vi "expt overnight automator set coils and save - arb coil patterns.vi"() -> ()   [LabVIEW 2018]
panel:
  in  "Save?":bool=TRUE
  in  "Field (Gauss)":u16(ring)=1 items=["9G"=1, "14G"=2]
  out "num coil iters done":i32
  out "total pos sweeps":i32
  out "total neg sweeps":i32
  in  "?":bool
  out "numSweeps list":i64[](array[numeric])=[10, 20, 10, 10, 20, 10]
  out "polarity list":i64[](array[numeric])=[-1, 1, -1, 1, -1, 1]
  in  "polarity pattern file":path=path "D:/rogers_data/GRA95229/115/thermal/115_s2_NWsulfide/TT_143C/P.txt"
  in  "num coil iterations":i32=2
  out "freq list (Hz)":dbl[](array[numeric])
  out "+Z current out (mA)":dbl=-975.0
  out "+Y current out (mA)":dbl=-1500.0
  out "+X current out (mA)":dbl=-20.0
  out "-Z current out (mA)":dbl=-975.0
  out "-Y current out (mA)":dbl=-1500.0
  out "-X current out (mA)":dbl=-20.0
  out "header cluster":T1
  in  "filename (adds .mat)":string="run_"
  in  "path":path=path "D:/rogers_data/GRA95229/115/thermal/115_s2_NWsulfide/TT_143C"
  out "coil polarity":bool=TRUE
  out "img data stack pos":dbl[][](array[numeric])
  in  "Height":i64(slide)=1200 min=0 max=1200 step=4 scale=0.0..1200.0
  in  "Width":i64(slide)=1920 min=0 max=1920 step=4 scale=0.0..1920.0
  out "img data stack neg":dbl[][](array[numeric])
  in  "freq range":T2(ring)=enum."Both ranges"
  in  "num freqs":i32=51
  out "set later end time!":bool
  out "current time":timestamp
  in  "end time (>current time)":timestamp=timestamp(3667924096.6668215 s since 1904-01-01)
  # "Coil parameters"
  # "Set time"
  # "Coil polarity"
  # "ODMR parameters"
  # "File setup"
  # "Camera parameters"
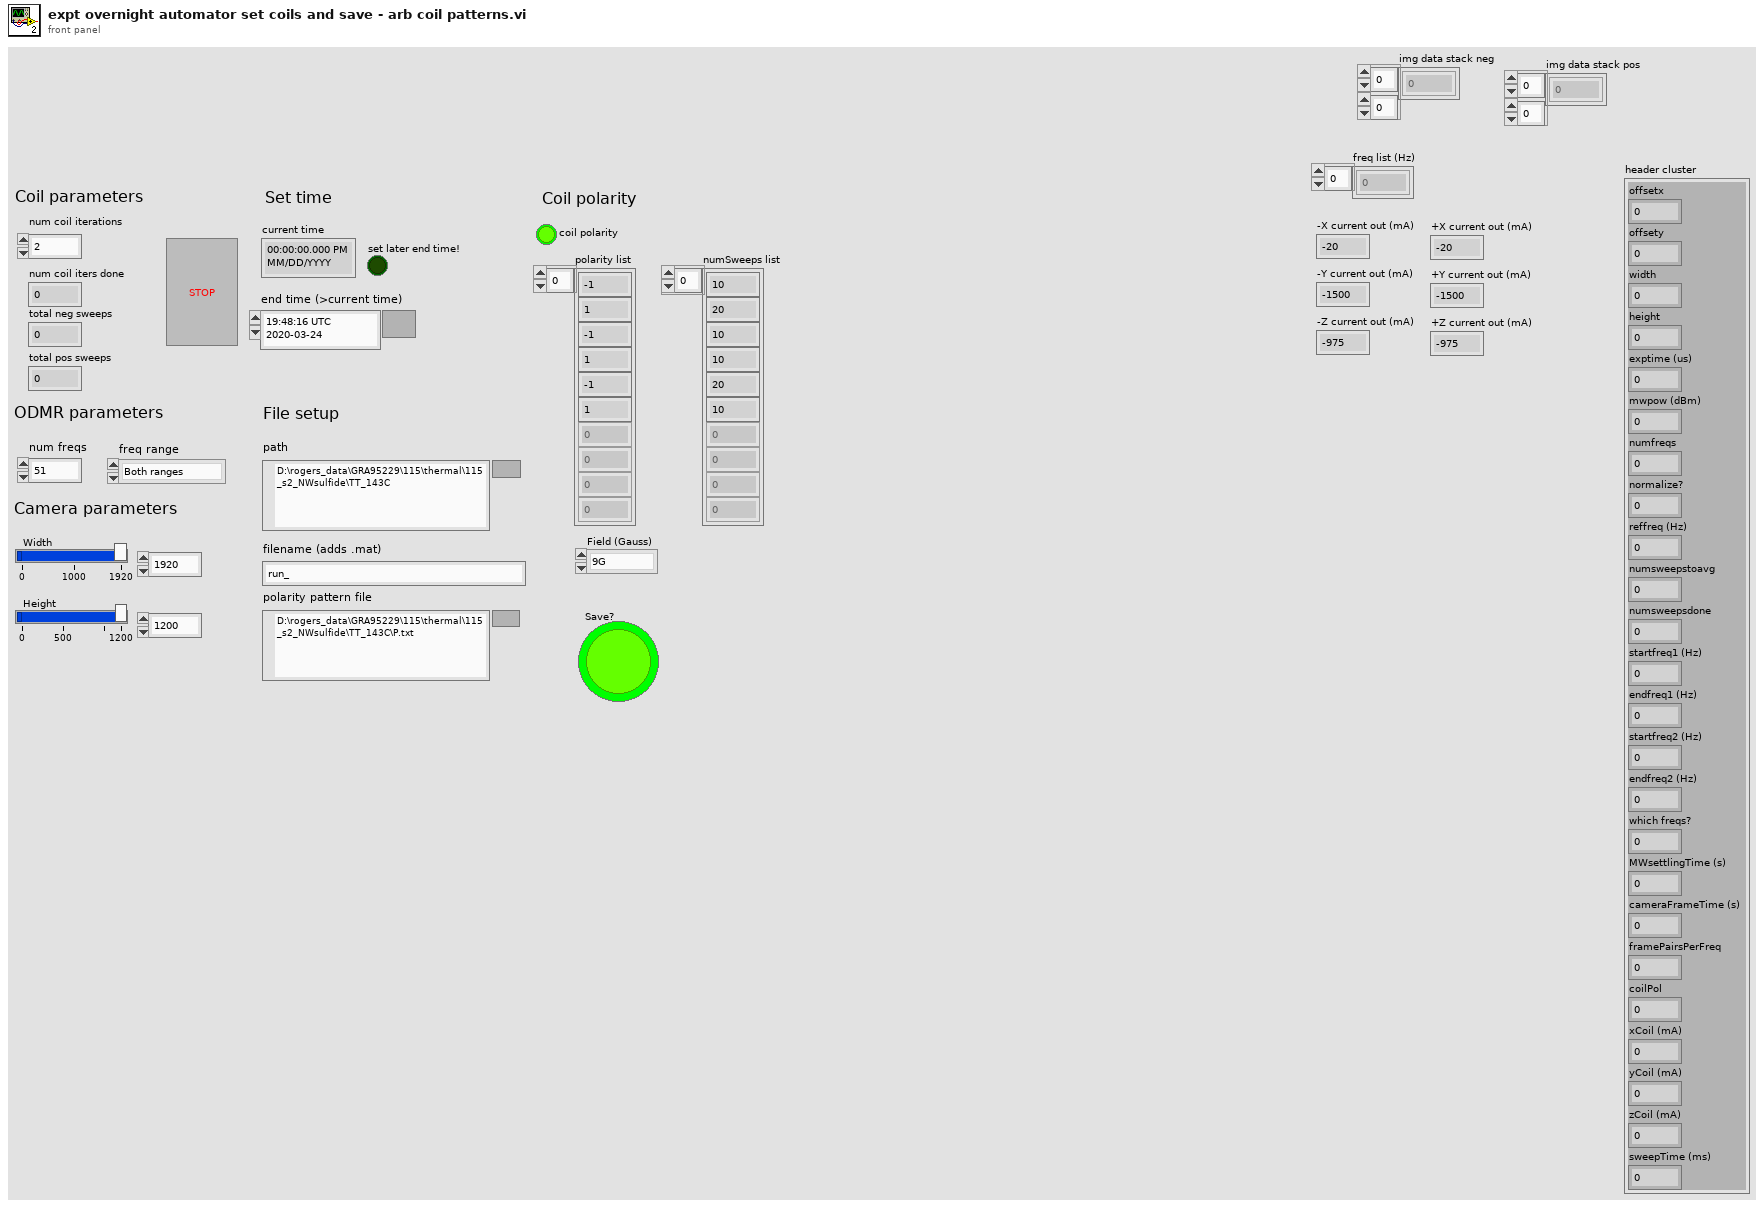
[diagram p1: front panel]
types:
  T1 = cluster{"offsetx":i64, "offsety":i64, "width":i64, "height":i64, "exptime (us)":dbl, "mwpow (dBm)":dbl, "numfreqs":i32, "normalize?":i32, "reffreq (Hz)":dbl, "numsweepstoavg":i32, "numsweepsdone":i32, "startfreq1 (Hz)":dbl, "endfreq1 (Hz)":dbl, "startfreq2 (Hz)":dbl, "endfreq2 (Hz)":dbl, "which freqs?":i32, "MWsettlingTime (s)":dbl, "cameraFrameTime (s)":dbl, "framePairsPerFreq":i32, "coilPol":i32, "xCoil (mA)":dbl, "yCoil (mA)":dbl, "zCoil (mA)":dbl, "sweepTime (ms)":i32}
  T2 = enum16{"Lower range", "Upper range", "Both ranges"}
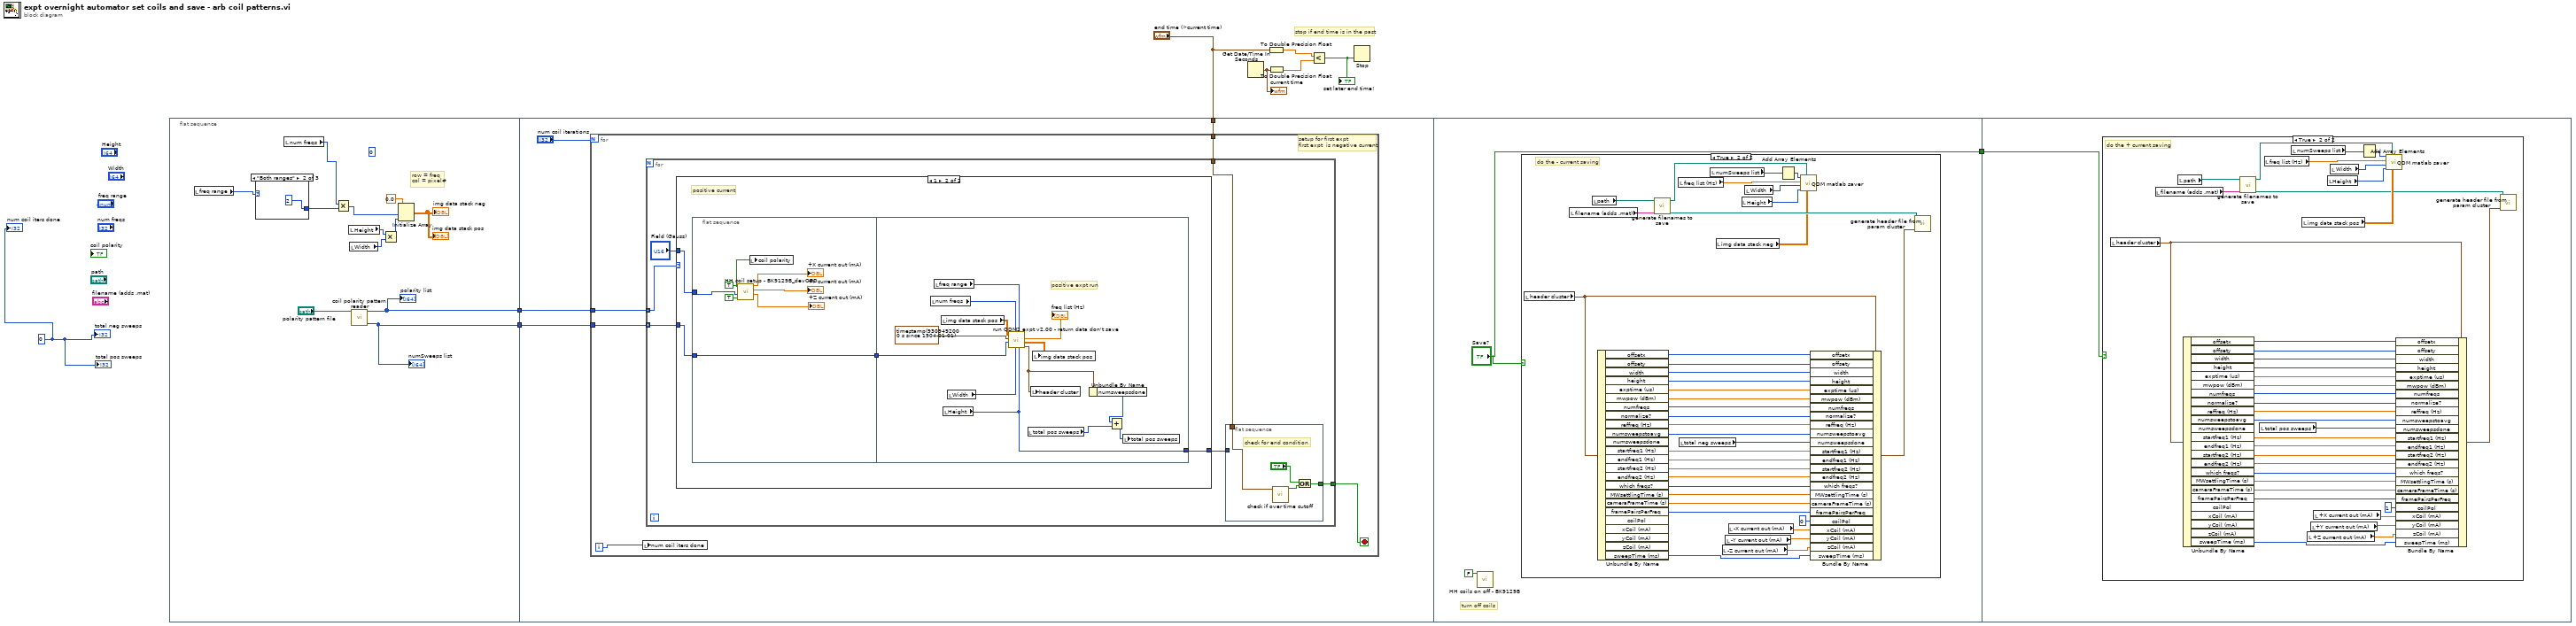
[diagram p0: block diagram]
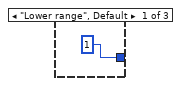
[diagram p2: hidden frame]
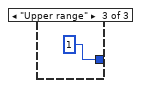
[diagram p3: hidden frame]
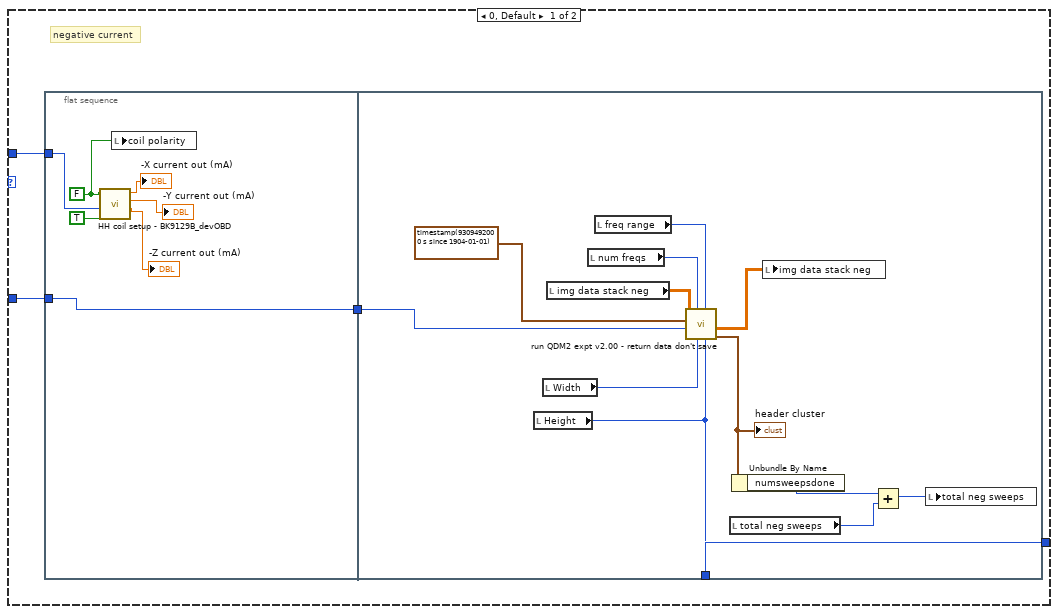
[diagram p4: hidden frame]
diagram:
  w2 = 0
  # "stop if end time is in the past"
  n1 = flat-sequence {
    tunnel: [w11] -> w9
    tunnel: [w10] -> w8
    tunnel: w9 -> [w28]
    tunnel: w8 -> [w27]
    tunnel: "end time (>current time)" -> [w25]
    tunnel: ["Save?"] -> w1
    tunnel: w1 -> [w129]
    frame #0 {
      (unwired) 0 ("1st half sweeps")
      # "row = freq\ncol = pixel#"
      n2 = local read "freq range"() -> (w13:T2)
      n3 = case shown="\"Both ranges\"" w13 {
        tunnel: [1 ("numFreqs") 2 ("numFreqs") 1 ("numFreqs")] -> w16
        frame "Lower range", Default {
        }
        frame "Both ranges" {
        }
        frame "Upper range" {
        }
      }
      n4 = local read "num freqs"() -> (w14:i32)
      n5 = Multiply(x=w14, y=w16) -> (x*y=w15:i32)
      n6 = local read "Height"() -> (w21:i64)
      n7 = local read "Width"() -> (w20:i64)
      n8 = call "coil polarity pattern reader.vi"("polarity pattern file"="polarity pattern file") -> ("numSweeps list"=w10:i64[], "polarity list"=w11:i64[])  [unwired: 9 in]
      "polarity list" <- w11
      "numSweeps list" <- w10
      n9 = Multiply(x=w21, y=w20) -> (x*y=w19:i64)
      n10 = Initialize Array(0.0 ("element"), w15, w19) -> (→"img data stack pos" →"img data stack neg":dbl[][])
    }
    frame #1 {
      n11 = for {
        N: "num coil iterations" -> [_]
        tunnel: w28 -> [w33]
        tunnel: w27 -> [w32]
        tunnel: w25 -> [w30]
        i -> [w29]
        stop <- w31 stop-if-true
        # "setup for first expt\nfirst expt  is negative current"
        n12 = local write "num coil iters done"(w29) -> ()
        n13 = for {
          tunnel: w33 -> [w39] mode=indexing
          tunnel: w32 -> [w38] mode=indexing
          tunnel: [w36] -> w31
          tunnel: w30 -> [w35]
          n14 = case shown="1" w39 {
            tunnel: w38 -> [w46 w70]
            tunnel: [w45 w68] -> w37
            tunnel: "Field (Gauss)" -> [w44 w67]
            frame 0, Default {
              # "negative current"
              n15 = flat-sequence {
                tunnel: [w54] -> w47
                tunnel: w46 -> [w54]
                tunnel: w44 -> [w48]
                tunnel: w47 -> [w61]
                tunnel: [w59] -> w45
                frame #0 {
                  w53 = FALSE ("coil polarity")
                  n16 = call "HH coil setup - BK9129B_devOBD.VI"("setup enabled?"=TRUE, "number"=w48, "coil polarity"=w53) -> ("Z current out (mA)"=→"-Z current out (mA)":dbl, "Y current out (mA)"=→"-Y current out (mA)":dbl, "X current out (mA)"=→"-X current out (mA)":dbl)  [unwired: 6 in]
                  n17 = local write "coil polarity"(w53) -> ()
                }
                frame #1 {
                  n18 = local read "Height"() -> (w59:i64)
                  n19 = local read "Width"() -> (w64:i64)
                  n20 = local read "img data stack neg"() -> (w62:dbl[][])
                  n21 = local read "num freqs"() -> (w66:i32)
                  n22 = local read "freq range"() -> (w65:T2)
                  n23 = call "run QDM2 expt v2.00 - return data don't save.vi"("Height"=w59, "which freqs?"=w65, "Width"=w64, "numFreqs"=w66, "num sweeps to avg"=w61, "cutoff time"=timestamp(9309492000 s since 1904-01-01), "img data stack Input"=w62) -> ("header cluster"=w58:T1, "img data stack Return"=w63:dbl[][])  [unwired: 1 in, 2 out]
                  "header cluster" <- w58
                  n24 = local read "total neg sweeps"() -> (w56:i32)
                  n25 = Unbundle By Name(w58) -> ("numsweepsdone"=w57:i32)
                  n26 = local write "img data stack neg"(w63) -> ()
                  n27 = Add(x=w57, y=w56) -> (x+y=w55:i32)
                  n28 = local write "total neg sweeps"(w55) -> ()
                }
              }
            }
            frame 1 {
              # "positive current"
              n29 = flat-sequence {
                tunnel: w70 -> [w72]
                tunnel: [w72] -> w69
                tunnel: w67 -> [w71]
                tunnel: w69 -> [w83]
                tunnel: [w82] -> w68
                frame #0 {
                  w73 = TRUE ("coil polarity")
                  n30 = call "HH coil setup - BK9129B_devOBD.VI"("setup enabled?"=TRUE, "number"=w71, "coil polarity"=w73) -> ("Z current out (mA)"=→"+Z current out (mA)":dbl, "Y current out (mA)"=→"+Y current out (mA)":dbl, "X current out (mA)"=→"+X current out (mA)":dbl)  [unwired: 6 in]
                  n31 = local write "coil polarity"(w73) -> ()
                }
                frame #1 {
                  # "positive expt run"
                  n32 = local read "num freqs"() -> (w90:i32)
                  n33 = local read "freq range"() -> (w89:T2)
                  n34 = local read "img data stack pos"() -> (w85:dbl[][])
                  n35 = local read "Height"() -> (w82:i64)
                  n36 = local read "Width"() -> (w88:i64)
                  n37 = call "run QDM2 expt v2.00 - return data don't save.vi"("Height"=w82, "which freqs?"=w89, "Width"=w88, "numFreqs"=w90, "num sweeps to avg"=w83, "cutoff time"=timestamp(9309492000 s since 1904-01-01), "img data stack Input"=w85) -> ("header cluster"=w81:T1, "img data stack Return"=w86:dbl[][], "freq list (Hz)"=→"freq list (Hz)":dbl[])  [unwired: 1 in, 1 out]
                  n38 = local read "total pos sweeps"() -> (w79:i32)
                  n39 = local write "header cluster"(w81) -> ()
                  n40 = local write "img data stack pos"(w86) -> ()
                  n41 = Unbundle By Name(w81) -> ("numsweepsdone"=w80:i32)
                  n42 = Add(x=w80, y=w79) -> (x+y=w78:i32)
                  n43 = local write "total pos sweeps"(w78) -> ()
                }
              }
            }
          }
          n44 = flat-sequence {
            tunnel: w37 -> [_]
            tunnel: [w41] -> w36
            tunnel: w35 -> [w40]
            frame #0 {
              # "check for end condition"
              n45 = call "check if over time cutoff.vi"("cutoff time"=w40) -> ("past due?"=w42:bool)  [unwired: 10 in]
              n46 = Or(x="?", y=w42) -> (x .or. y?=w41:bool)
            }
          }
        }
      }
    }
    frame #2 {
      # "turn off coils"
      n47 = call "HH coils on off - BK9129B.VI"("coils on?"=FALSE) -> ()  [unwired: 11 in]
      n48 = case shown="True" "Save?" {
        frame False {
        }
        frame True {
          # "do the - current saving"
          n49 = local read "header cluster"() -> (w103:T1)
          n50 = local read "filename (adds .mat)"() -> (w127:string)
          n51 = local read "path"() -> (w128:path)
          n52 = Unbundle By Name(w103) -> ("offsetx"=w104:i64, "offsety"=w105:i64, "width"=w106:i64, "height"=w107:i64, "exptime (us)"=w108:dbl, "mwpow (dBm)"=w109:dbl, "numfreqs"=w110:i32, "normalize?"=w111:i32, "reffreq (Hz)"=w112:dbl, "numsweepstoavg"=w113:i32, "startfreq1 (Hz)"=w114:dbl, "endfreq1 (Hz)"=w115:dbl, "startfreq2 (Hz)"=w116:dbl, "endfreq2 (Hz)"=w117:dbl, "which freqs?"=w118:i32, "MWsettlingTime (s)"=w119:dbl, "cameraFrameTime (s)"=w120:dbl, "framePairsPerFreq"=w121:i32, "sweepTime (ms)"=w122:i32)  [unwired: 5 out]
          n53 = call "generate filenames to save.vi"("filename (adds .mat)"=w127, "path"=w128) -> ("header path"=w126:path, "matlab path"=w101:path)  [unwired: 8 in]
          n54 = local read "freq list (Hz)"() -> (w97:dbl[])
          n55 = local read "total neg sweeps"() -> (w93:i32)
          n56 = local read "numSweeps list"() -> (w95:i64[])
          n57 = local read "img data stack neg"() -> (w98:dbl[][])
          n58 = local read "-Z current out (mA)"() -> (w125:dbl)
          n59 = local read "-Y current out (mA)"() -> (w124:dbl)
          n60 = local read "-X current out (mA)"() -> (w123:dbl)
          n61 = local read "Height"() -> (w99:i64)
          n62 = local read "Width"() -> (w100:i64)
          n63 = Add Array Elements(numeric array=w95) -> (sum=w94:i64)
          n64 = call "QDM matlab saver.vi"("img data stack Input"=w98, "matlab path"=w101, "Height"=w99, "Width"=w100, "freq list (Hz)"=w97, "sweep #"=w94) -> ()  [unwired: 6 in]
          n65 = Bundle By Name(cluster=w103, "offsetx"=w104, "offsety"=w105, "width"=w106, "height"=w107, "exptime (us)"=w108, "mwpow (dBm)"=w109, "numfreqs"=w110, "normalize?"=w111, "reffreq (Hz)"=w112, "numsweepstoavg"=w113, "numsweepsdone"=w93, "startfreq1 (Hz)"=w114, "endfreq1 (Hz)"=w115, "startfreq2 (Hz)"=w116, "endfreq2 (Hz)"=w117, "which freqs?"=w118, "MWsettlingTime (s)"=w119, "cameraFrameTime (s)"=w120, "framePairsPerFreq"=w121, "coilPol"=0, "xCoil (mA)"=w123, "yCoil (mA)"=w124, "zCoil (mA)"=w125, "sweepTime (ms)"=w122) -> (w102:T1)
          n66 = call "generate header file from param cluster.vi"("output cluster"=w102, "header path (full)"=w126) -> ()  [unwired: 10 in]
        }
      }
    }
    frame #3 {
      n67 = case shown="True" w129 {
        frame False {
        }
        frame True {
          # "do the + current saving"
          n68 = local read "header cluster"() -> (w159:T1)
          n69 = local read "filename (adds .mat)"() -> (w135:string)
          n70 = local read "path"() -> (w134:path)
          n71 = Unbundle By Name(w159) -> ("offsetx"=w158:i64, "offsety"=w157:i64, "width"=w156:i64, "height"=w155:i64, "exptime (us)"=w154:dbl, "mwpow (dBm)"=w153:dbl, "numfreqs"=w152:i32, "normalize?"=w151:i32, "reffreq (Hz)"=w150:dbl, "numsweepstoavg"=w149:i32, "startfreq1 (Hz)"=w148:dbl, "endfreq1 (Hz)"=w147:dbl, "startfreq2 (Hz)"=w146:dbl, "endfreq2 (Hz)"=w145:dbl, "which freqs?"=w144:i32, "MWsettlingTime (s)"=w143:dbl, "cameraFrameTime (s)"=w142:dbl, "framePairsPerFreq"=w141:i32, "sweepTime (ms)"=w140:i32)  [unwired: 5 out]
          n72 = call "generate filenames to save.vi"("filename (adds .mat)"=w135, "path"=w134) -> ("header path"=w136:path, "matlab path"=w161:path)  [unwired: 8 in]
          n73 = local read "total pos sweeps"() -> (w130:i32)
          n74 = local read "freq list (Hz)"() -> (w165:dbl[])
          n75 = local read "numSweeps list"() -> (w132:i64[])
          n76 = local read "img data stack pos"() -> (w164:dbl[][])
          n77 = local read "+Z current out (mA)"() -> (w137:dbl)
          n78 = local read "+Y current out (mA)"() -> (w138:dbl)
          n79 = local read "+X current out (mA)"() -> (w139:dbl)
          n80 = local read "Height"() -> (w163:i64)
          n81 = local read "Width"() -> (w162:i64)
          n82 = Add Array Elements(numeric array=w132) -> (sum=w131:i64)
          n83 = call "QDM matlab saver.vi"("img data stack Input"=w164, "matlab path"=w161, "Height"=w163, "Width"=w162, "freq list (Hz)"=w165, "sweep #"=w131) -> ()  [unwired: 6 in]
          n84 = Bundle By Name(cluster=w159, "offsetx"=w158, "offsety"=w157, "width"=w156, "height"=w155, "exptime (us)"=w154, "mwpow (dBm)"=w153, "numfreqs"=w152, "normalize?"=w151, "reffreq (Hz)"=w150, "numsweepstoavg"=w149, "numsweepsdone"=w130, "startfreq1 (Hz)"=w148, "endfreq1 (Hz)"=w147, "startfreq2 (Hz)"=w146, "endfreq2 (Hz)"=w145, "which freqs?"=w144, "MWsettlingTime (s)"=w143, "cameraFrameTime (s)"=w142, "framePairsPerFreq"=w141, "coilPol"=1, "xCoil (mA)"=w139, "yCoil (mA)"=w138, "zCoil (mA)"=w137, "sweepTime (ms)"=w140) -> (w160:T1)
          n85 = call "generate header file from param cluster.vi"("output cluster"=w160, "header path (full)"=w136) -> ()  [unwired: 10 in]
        }
      }
    }
  }
  n86 = Get Date/Time In Seconds() -> (seconds since 1Jan1904=w7:timestamp)
  "current time" <- w7
  n87 = To Double Precision Float(number="end time (>current time)") -> (double precision float=w6:dbl)
  n88 = To Double Precision Float(number=w7) -> (double precision float=w5:dbl)
  n89 = Less?(x=w6, y=w5) -> (x < y?=w4:bool)
  "set later end time!" <- w4
  n90 = Stop(stop? (T)=w4) -> ()
  "total neg sweeps" <- w2
  "total pos sweeps" <- w2
  "num coil iters done" <- w2
